vi "Configure Sweep.vi"(7 "Sweep Mode (0: Chopped)":i32(ring) items=["Chopped", "Alternate"], 8 "error in (no error)":errorcluster, 9 "Sweep Type (0: Linear)":i32(ring) items=["Linear", "Logarithmic", "Power", "CW", "Segment", "Phase"], 10 "Channel (1)":i32=1, 11 "VISA resource name":refnum<visa-resource-name>) -> (0 "error out":errorcluster, 3 "VISA resource name out":refnum<visa-resource-name>)   [LabVIEW 2018, in "Keysight PNA Series.lvlib"]
doc: "Configures sweep."
uses:
  Keysight PNA Series.lvlib
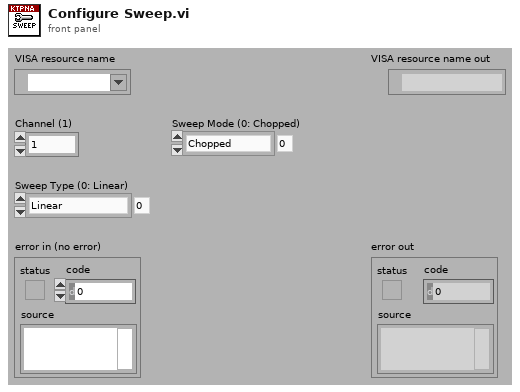
[diagram p1: front panel]
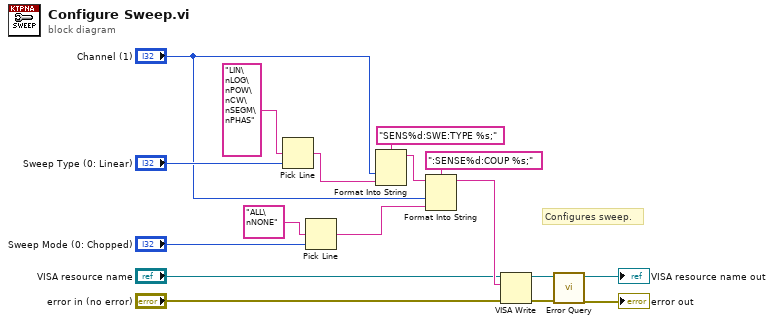
[diagram p0: block diagram]
diagram:
  # "Configures sweep."
  n1 = Pick Line(multi-line string="LIN\nLOG\nPOW\nCW\nSEGM\nPHAS", line index="Sweep Type (0: Linear)") -> (output string=w13:string)  [unwired: 1 in]
  n2 = Pick Line(multi-line string="ALL\nNONE", line index="Sweep Mode (0: Chopped)") -> (output string=w8:string)  [unwired: 1 in]
  n3 = Format Into String(format string="SENS%d:SWE:TYPE %s;", "Channel (1)", w13) -> (resulting string=w10:string)  [unwired: 2 in, 1 out]
  n4 = Format Into String(format string=":SENSE%d:COUP %s;", initial string=w10, "Channel (1)", w8) -> (resulting string=w7:string)  [unwired: 1 in, 1 out]
  n5 = VISA Write(VISA resource name="VISA resource name", write buffer=w7, error in (no error)="error in (no error)") -> (VISA resource name out=w4:refnum<visa-resource-name>, error out=w3:errorcluster)  [unwired: 1 out]
  n6 = call "Error Query.vi"("error in (no error)"=w3, "VISA resource name"=w4) -> ("error out"=→"error out":errorcluster, "VISA resource name out"=→"VISA resource name out":refnum<visa-resource-name>)  [unwired: 6 in, 2 out]
